vi "example_asynch_wait_example.vi"() -> ()   [LabVIEW 2015]
uses:
  polys/poly_now_ms_timer.vi
  polys/poly_asynch_wait_wait.vi
  cores/core_timing_tools_eco.vi
  polys/poly_timing_tools_eco_plus.vi
  ref_tools/name_of_caller.vi
  <vilib>/Utility/error.llb/Clear Errors.vi
  polys/poly_asynch_wait_start.vi
  polys/poly_asynch_wait_notify.vi
  polys/poly_asynch_wait_stop.vi
  error_tools/toolbox_error_handler.vi
  <vilib>/Utility/error.llb/Simple Error Handler.vi
  loop_timeout.vi
  polys/poly_loop_timeout_bool.vi
panel:
  out "4 wait time":u32
  out "3 wait time":u32
  out "2 wait time":u32
  out "1 wait time":u32
  in  "stop":bool
  out "4 refnum":u32
  out "3 refnum":u32
  out "2 refnum":u32
  out "1 refnum":u32
  in  "4 stop":bool
  in  "3 stop":bool
  in  "2 stop":bool
  in  "4 notify":bool
  in  "3 notify":bool
  in  "2 notify":bool
  in  "4 timeout":i32=-1 format="%.0f ms"
  in  "3 timeout":i32=3000 format="%.0f ms"
  in  "2 timeout":i32=2000 format="%.0f ms"
  in  "1 timeout":i32=1000 format="%.0f ms"
  in  "1 stop":bool
  in  "1 notify":bool
  out "4 error":bool
  out "3 error":bool
  out "2 error":bool
  out "1 error":bool
  out "4 timeout":bool
  out "3 timeout":bool
  out "2 timeout":bool
  out "1 tiemout":bool
  out "4 done":bool
  out "3 done":bool
  out "2 done":bool
  out "1 done":bool
  # "notifier refnum"
  # "timeout [ms]"
  # "done"
  # "timed out"
  # "error"
  # "send notif."
  # "send notif."
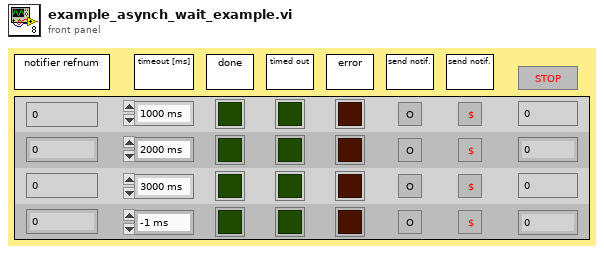
[diagram p1: front panel]
types:
  T1 = typedef "boolean_notifier2.ctl" = refnum<queue>
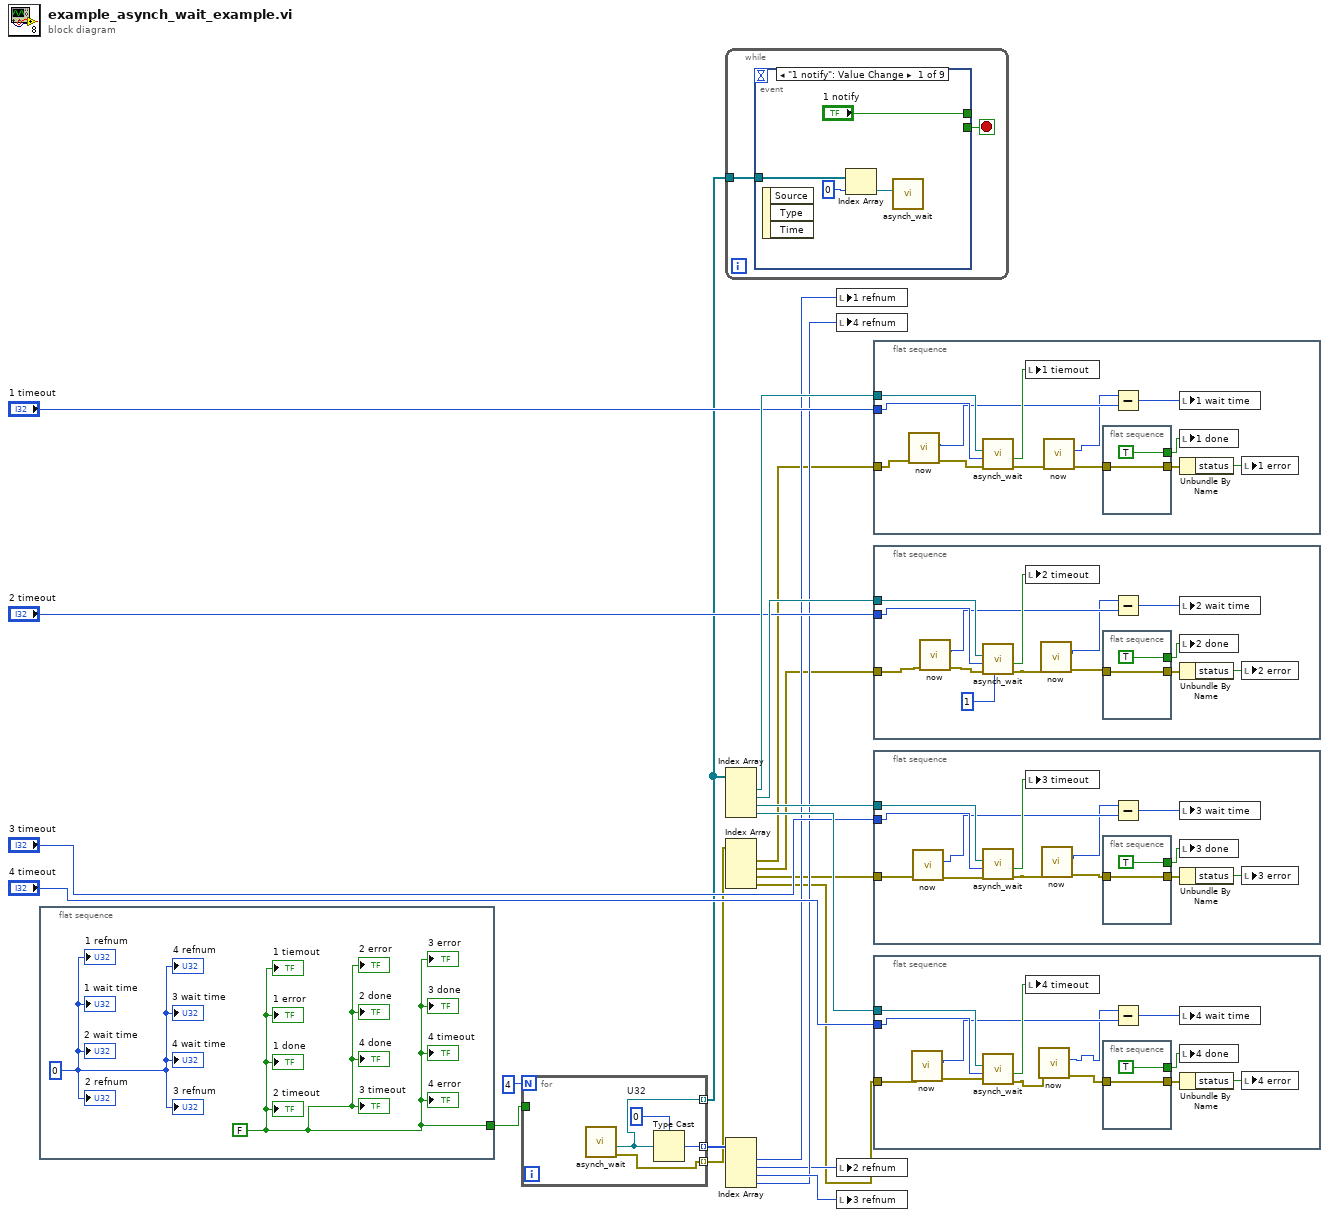
[diagram p0: block diagram]
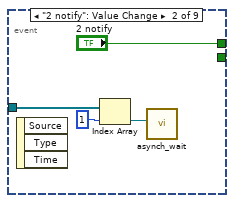
[diagram p2: hidden frame]
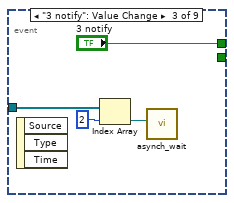
[diagram p3: hidden frame]
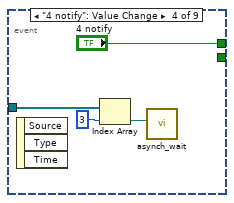
[diagram p4: hidden frame]
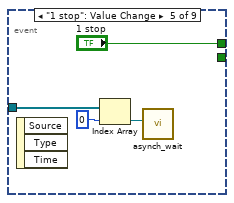
[diagram p5: hidden frame]
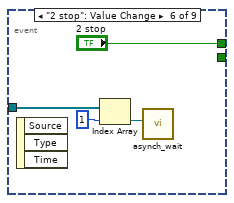
[diagram p6: hidden frame]
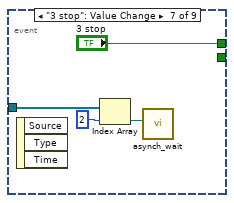
[diagram p7: hidden frame]
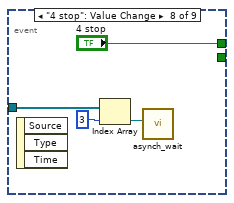
[diagram p8: hidden frame]
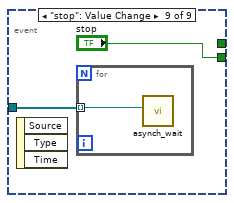
[diagram p9: hidden frame]
diagram:
  n1 = flat-sequence {
    tunnel: [w22] -> w17
    frame #0 {
      w22 = FALSE
      w23 = u32 0
      "1 done" <- w22
      "2 done" <- w22
      "3 done" <- w22
      "4 done" <- w22
      "1 tiemout" <- w22
      "2 timeout" <- w22
      "3 timeout" <- w22
      "4 timeout" <- w22
      "1 error" <- w22
      "2 error" <- w22
      "3 error" <- w22
      "4 error" <- w22
      "1 refnum" <- w23
      "2 refnum" <- w23
      "3 refnum" <- w23
      "4 refnum" <- w23
      "1 wait time" <- w23
      "2 wait time" <- w23
      "3 wait time" <- w23
      "4 wait time" <- w23
    }
  }
  n2 = for {
    N: 4 -> [_]
    tunnel: [w26] -> w11 mode=indexing
    tunnel: [w24] -> w10 mode=indexing
    tunnel: w17 -> [_]
    tunnel: [w25] -> w5 mode=indexing
    w27 = u32 0  # U32
    n3 = call-poly "asynch_wait.vi"() -> ("error out"=w25:errorcluster, "notifier"=w24:T1)  [unwired: 9 in, 1 out]
    n4 = Type Cast(type=w27, x=w24) -> (*(type *) &x=w26:u32)
  }
  n5 = while {
    tunnel: w10 -> [w29]
    stop <- w28 stop-if-true
    n6 = event shown="[0] \"1 notify\": Value Change" {
      selector: _ -> [_ _ _ _ _ _ _ _ _]
      dyn-events: _ -> [_ _ _ _ _ _ _ _ _]
      timeout: _ -> [_ _ _ _ _ _ _ _ _]
      tunnel: w29 -> [w33 w37 w41 w45 w49 w53 w57 w61 w62]
      tunnel: ["1 notify" "2 notify" "3 notify" "4 notify" "1 stop" "2 stop" "3 stop" "4 stop" _] -> _
      tunnel: [_ _ _ _ _ _ _ _ "stop"] -> w28
      event "1 notify": Value Change {
        n7 = event-data() -> ()  [unwired: 1 in, 3 out]
        n8 = Index Array(array=w33, index=0) -> (element=w30:T1)
        n9 = call-poly "asynch_wait.vi"("notifier"=w30) -> ()  [unwired: 10 in, 1 out]
      }
      event "2 notify": Value Change {
        n10 = event-data() -> ()  [unwired: 1 in, 3 out]
        n11 = Index Array(array=w37, index=1) -> (element=w34:T1)
        n12 = call-poly "asynch_wait.vi"("notifier"=w34) -> ()  [unwired: 10 in, 1 out]
      }
      event "3 notify": Value Change {
        n13 = event-data() -> ()  [unwired: 1 in, 3 out]
        n14 = Index Array(array=w41, index=2) -> (element=w38:T1)
        n15 = call-poly "asynch_wait.vi"("notifier"=w38) -> ()  [unwired: 10 in, 1 out]
      }
      event "4 notify": Value Change {
        n16 = event-data() -> ()  [unwired: 1 in, 3 out]
        n17 = Index Array(array=w45, index=3) -> (element=w42:T1)
        n18 = call-poly "asynch_wait.vi"("notifier"=w42) -> ()  [unwired: 10 in, 1 out]
      }
      event "1 stop": Value Change {
        n19 = event-data() -> ()  [unwired: 1 in, 3 out]
        n20 = Index Array(array=w49, index=0) -> (element=w47:T1)
        n21 = call-poly "asynch_wait.vi"("notifier"=w47) -> ()  [unwired: 10 in, 1 out]
      }
      event "2 stop": Value Change {
        n22 = event-data() -> ()  [unwired: 1 in, 3 out]
        n23 = Index Array(array=w53, index=1) -> (element=w51:T1)
        n24 = call-poly "asynch_wait.vi"("notifier"=w51) -> ()  [unwired: 10 in, 1 out]
      }
      event "3 stop": Value Change {
        n25 = event-data() -> ()  [unwired: 1 in, 3 out]
        n26 = Index Array(array=w57, index=2) -> (element=w55:T1)
        n27 = call-poly "asynch_wait.vi"("notifier"=w55) -> ()  [unwired: 10 in, 1 out]
      }
      event "4 stop": Value Change {
        n28 = event-data() -> ()  [unwired: 1 in, 3 out]
        n29 = Index Array(array=w61, index=3) -> (element=w59:T1)
        n30 = call-poly "asynch_wait.vi"("notifier"=w59) -> ()  [unwired: 10 in, 1 out]
      }
      event "stop": Value Change {
        n31 = event-data() -> ()  [unwired: 1 in, 3 out]
        n32 = for {
          tunnel: w62 -> [w64] mode=indexing
          n33 = call-poly "asynch_wait.vi"("notifier"=w64) -> ()  [unwired: 10 in, 1 out]
        }
      }
    }
  }
  n34 = Index Array(array=w10) -> (element #1=w20:T1, element #2=w19:T1, element #3=w18:T1, element #4=w16:T1)  [unwired: 4 in]
  n35 = Index Array(array=w5) -> (element #1=w4:errorcluster, element #2=w3:errorcluster, element #3=w2:errorcluster, element #4=w1:errorcluster)  [unwired: 4 in]
  n36 = Index Array(array=w11) -> (element #1=w9:u32, element #2=w6:u32, element #3=w8:u32, element #4=w7:u32)  [unwired: 4 in]
  n37 = local write "1 refnum"(w9) -> ()
  n38 = local write "4 refnum"(w7) -> ()
  n39 = local write "2 refnum"(w6) -> ()
  n40 = local write "3 refnum"(w8) -> ()
  n41 = flat-sequence {
    tunnel: w20 -> [w77]
    tunnel: "1 timeout" -> [w74]
    tunnel: w4 -> [w69]
    frame #0 {
      n42 = call-poly "now.vi"("Error in"=w69) -> ("Error out"=w68:errorcluster, "millisecond timer value"=w70:i32)  [unwired: 9 in]
      n43 = call-poly "asynch_wait.vi"("error in"=w68, "timeout"=w74, "notifier"=w77) -> ("error out"=w67:errorcluster, "timed out?"=w76:bool)  [unwired: 6 in, 1 out]
      n44 = local write "1 tiemout"(w76) -> ()
      n45 = call-poly "now.vi"("Error in"=w67) -> ("Error out"=w65:errorcluster, "millisecond timer value"=w66:i32)  [unwired: 9 in]
      n46 = flat-sequence {
        tunnel: [TRUE] -> w72
        tunnel: [w78] -> w73
        tunnel: w65 -> [w78]
        frame #0 {
        }
      }
      n47 = Subtract(x=w66, y=w70) -> (x-y=w71:i32)
      n48 = local write "1 wait time"(w71) -> ()
      n49 = local write "1 done"(w72) -> ()
      n50 = Unbundle By Name(w73) -> ("status"=w75:bool)
      n51 = local write "1 error"(w75) -> ()
    }
  }
  n52 = flat-sequence {
    tunnel: w19 -> [w93]
    tunnel: "2 timeout" -> [w90]
    tunnel: w3 -> [w86]
    frame #0 {
      n53 = call-poly "now.vi"("Error in"=w86) -> ("Error out"=w84:errorcluster, "millisecond timer value"=w85:i32)  [unwired: 9 in]
      n54 = call-poly "asynch_wait.vi"("check interval (50 ms)"=u32 1, "error in"=w84, "timeout"=w90, "notifier"=w93) -> ("error out"=w83:errorcluster, "timed out?"=w92:bool)  [unwired: 5 in, 1 out]
      n55 = local write "2 timeout"(w92) -> ()
      n56 = call-poly "now.vi"("Error in"=w83) -> ("Error out"=w81:errorcluster, "millisecond timer value"=w82:i32)  [unwired: 9 in]
      n57 = flat-sequence {
        tunnel: [TRUE] -> w88
        tunnel: [w94] -> w89
        tunnel: w81 -> [w94]
        frame #0 {
        }
      }
      n58 = Subtract(x=w82, y=w85) -> (x-y=w87:i32)
      n59 = local write "2 wait time"(w87) -> ()
      n60 = local write "2 done"(w88) -> ()
      n61 = Unbundle By Name(w89) -> ("status"=w91:bool)
      n62 = local write "2 error"(w91) -> ()
    }
  }
  n63 = flat-sequence {
    tunnel: w18 -> [w108]
    tunnel: "3 timeout" -> [w105]
    tunnel: w2 -> [w101]
    frame #0 {
      n64 = call-poly "now.vi"("Error in"=w101) -> ("Error out"=w100:errorcluster, "millisecond timer value"=w99:i32)  [unwired: 9 in]
      n65 = call-poly "asynch_wait.vi"("error in"=w100, "timeout"=w105, "notifier"=w108) -> ("error out"=w98:errorcluster, "timed out?"=w107:bool)  [unwired: 6 in, 1 out]
      n66 = local write "3 timeout"(w107) -> ()
      n67 = call-poly "now.vi"("Error in"=w98) -> ("Error out"=w96:errorcluster, "millisecond timer value"=w97:i32)  [unwired: 9 in]
      n68 = flat-sequence {
        tunnel: [TRUE] -> w103
        tunnel: [w109] -> w104
        tunnel: w96 -> [w109]
        frame #0 {
        }
      }
      n69 = Subtract(x=w97, y=w99) -> (x-y=w102:i32)
      n70 = local write "3 wait time"(w102) -> ()
      n71 = local write "3 done"(w103) -> ()
      n72 = Unbundle By Name(w104) -> ("status"=w106:bool)
      n73 = local write "3 error"(w106) -> ()
    }
  }
  n74 = flat-sequence {
    tunnel: w16 -> [w120]
    tunnel: "4 timeout" -> [w119]
    tunnel: w1 -> [w116]
    frame #0 {
      n75 = call-poly "now.vi"("Error in"=w116) -> ("Error out"=w115:errorcluster, "millisecond timer value"=w114:i32)  [unwired: 9 in]
      n76 = call-poly "asynch_wait.vi"("error in"=w115, "timeout"=w119, "notifier"=w120) -> ("error out"=w113:errorcluster, "timed out?"=w122:bool)  [unwired: 6 in, 1 out]
      n77 = local write "4 timeout"(w122) -> ()
      n78 = call-poly "now.vi"("Error in"=w113) -> ("Error out"=w112:errorcluster, "millisecond timer value"=w111:i32)  [unwired: 9 in]
      n79 = flat-sequence {
        tunnel: [TRUE] -> w123
        tunnel: [w124] -> w118
        tunnel: w112 -> [w124]
        frame #0 {
        }
      }
      n80 = Subtract(x=w111, y=w114) -> (x-y=w117:i32)
      n81 = local write "4 wait time"(w117) -> ()
      n82 = local write "4 done"(w123) -> ()
      n83 = Unbundle By Name(w118) -> ("status"=w121:bool)
      n84 = local write "4 error"(w121) -> ()
    }
  }
